vi "Write CSV File_2D.vi"(7 "delimiter (,)":string=",", 8 "error in (no error)":errorcluster, 9 "append to file? (new file)":bool, 10 "2D array":string[][](array[string]), 11 "file path in":path) -> (0 "error out":errorcluster, 3 "file path out":path)   [LabVIEW 2013, in "Robust CSV.lvlib"]
doc: "Write a 2D array of strings to CSV file. The CSV file is formatted in accordance with RFC-4180 (see http://tools.ietf.org/html/rfc4180). \n\nA custom delimiter character can be specified. Default is a comma.\n\nSetting \"append to file?\" to true will append the data to the end of an existing file. Setting \"append to file?\" to false will overwrite an existing file. In both cases, if the file is not found, a new file will be created.\n\nRev 0.0 2014-02-20 Ryan Porter\n- First Draft\n\nRev 0.1 2014-10-30 Ryan Porter\n- Removed \"Convert EOL\" option from write to file to preserve compatibility with Excel CSV import."
uses:
  Robust CSV.lvlib
panel:
  # "Write CSV File_2D.vi\n\nWrite a 2D array of strings to CSV file. The CSV file is formatted in accordance with RFC-4180 (see http://tools.ietf.org/html/rfc4180). \n\nA custom delimiter character can be specified. Default is a comma.\n\nSetting \"append to file?\" to true will append the data to the end of an existing file. Setting \"append to file?\" to false will overwrite an existing file. In both cases, if the file is not found, a new file will be created."
  # "License: BSD (2-Clause) - http://opensource.org/licenses/BSD-2-Clause \n\nCopyright (c) 2014, Ryan Porter\nAll rights reserved."
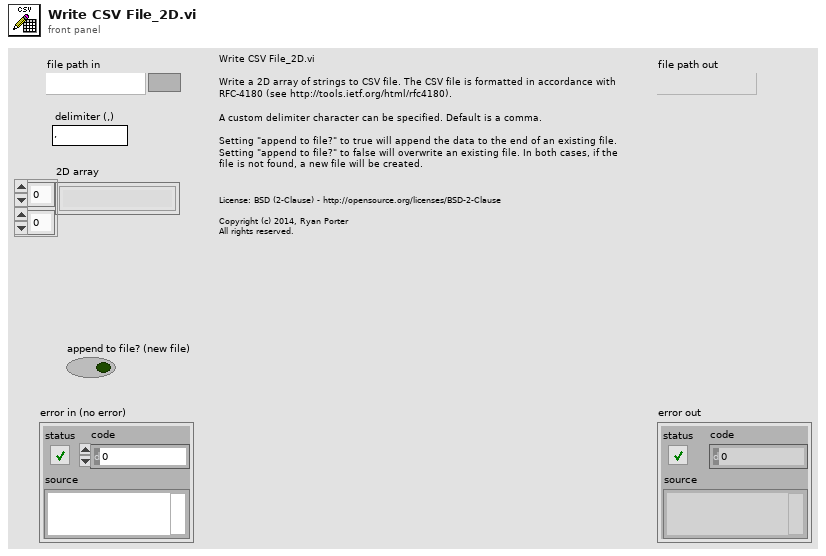
[diagram p1: front panel]
types:
  T1 = enum16{"open", "replace", "create", "open or create", "replace or create", "replace or create with confirmation"}
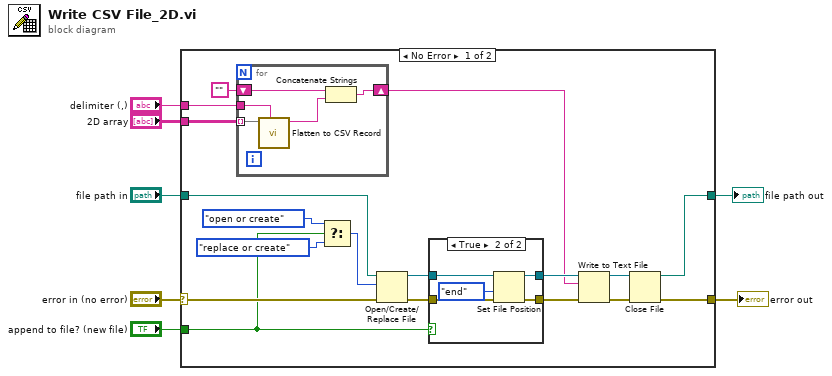
[diagram p0: block diagram]
diagram:
  n1 = case shown="No Error" "error in (no error)" {
    selector: "error in (no error)" -> [w22 w39]
    tunnel: "2D array" -> [w25 _]
    tunnel: "delimiter (,)" -> [w23 _]
    tunnel: [w11 w39] -> w4
    tunnel: "file path in" -> [w21 w38]
    tunnel: "append to file? (new file)" -> [w13 _]
    tunnel: [w8 w38] -> w1
    frame No Error {
      n2 = for {
        tunnel: w25 -> [w35] mode=indexing
        shift-right: [w36] -> w9
        shift-left: "" -> [w37]
        tunnel: w23 -> [w34]
        n3 = call "Flatten to CSV Record.vi"("delimiter (,)"=w34, "row of strings"=w35) -> ("CSV record"=w33:string)  [unwired: 8 in, 1 out]
        n4 = Concatenate Strings(w37, w33) -> (w36:string)
      }
      n5 = Select(t=T1."open or create" ("operation (0:open)"), s=w13, f=T1."replace or create" ("operation (0:open)")) -> (s? t:f=w18:T1)
      n6 = Open/Create/Replace File(file path (use dialog)=w21, error in=w22, operation (0:open)=w18) -> (refnum out=w17:refnum<file>, error out=w16:errorcluster)  [unwired: 3 in, 1 out]
      n7 = case shown="True" w13 {
        tunnel: w17 -> [w27 w32]
        tunnel: w16 -> [w26 w31]
        tunnel: [w26 w29] -> w15
        tunnel: [w27 w28] -> w14
        frame False {
        }
        frame True {
          n8 = Set File Position(refnum=w32, from (0:start)=enum16{"start", "end", "current"}."end", error in=w31) -> (refnum out=w28:refnum<file>, error out=w29:errorcluster)  [unwired: 1 in]
        }
      }
      n9 = Write to Text File(file (use dialog)=w14, text=w9, error in=w15) -> (refnum out=w10:refnum<file>, error out=w12:errorcluster)  [unwired: 1 in, 1 out]
      n10 = Close File(refnum=w10, error in=w12) -> (path=w8:path, error out=w11:errorcluster)
    }
    frame Error {
    }
  }
  "error out" <- w4
  "file path out" <- w1
